vi "DSF.Transceiver.UDP.Tx.vi"(8 "error in (no error)":errorcluster, 9 "Tx":T1, 11 "UDP Transceiver in":refnum<class "DSF.Transceiver.UDP.lvclass">=refnum) -> (0 "error out":errorcluster, 3 "UDP Transceiver out":refnum<class "DSF.Transceiver.UDP.lvclass">)   [LabVIEW 2017, in "DSF.Transceiver.UDP.lvlib" / "DSF.Transceiver.UDP.lvclass"]
uses:
  DSF.Transceiver.UDP.lvclass
  Builds/Current/Data Sharing Framework Core/Data Sharing Framework Core.lvlibp/Engine/Transfer/Transfer.lvclass
  Builds/Current/Data Sharing Framework Core/Data Sharing Framework Core.lvlibp/Engine/Internal/Memory/Memory Buffer/Memory Buffer.lvclass
  Builds/Current/Data Sharing Framework Core/Data Sharing Framework Core.lvlibp/Engine/Internal/Memory/Memory Buffer/Read 1D Array of U8.vi
  DSF.Transceiver.UDP.Parameters.Transfer.Tx.ctl
  DSF.Transceiver.UDP.Parameters.Transfer Group.Tx.ctl
panel:
  in  "Transfers":refnum<class "Transfer.lvclass">[](array[class])
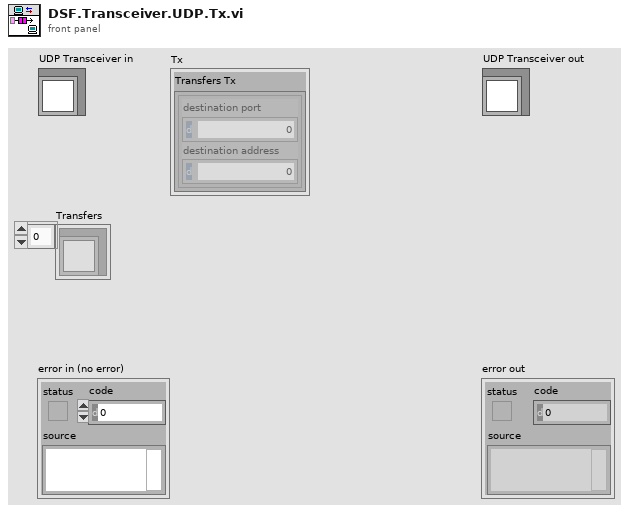
[diagram p1: front panel]
types:
  T1 = typedef "DSF.Transceiver.UDP.lvlib/DSF.Transceiver.UDP.lvclass/DSF.Transceiver.UDP.Parameters.Transfer Group.Tx.ctl" = cluster{"Transfers Tx":T2[]}
  T2 = typedef "DSF.Transceiver.UDP.lvlib/DSF.Transceiver.UDP.lvclass/DSF.Transceiver.UDP.Parameters.Transfer.Tx.ctl" = cluster{"destination port":u16, "destination address":u32}
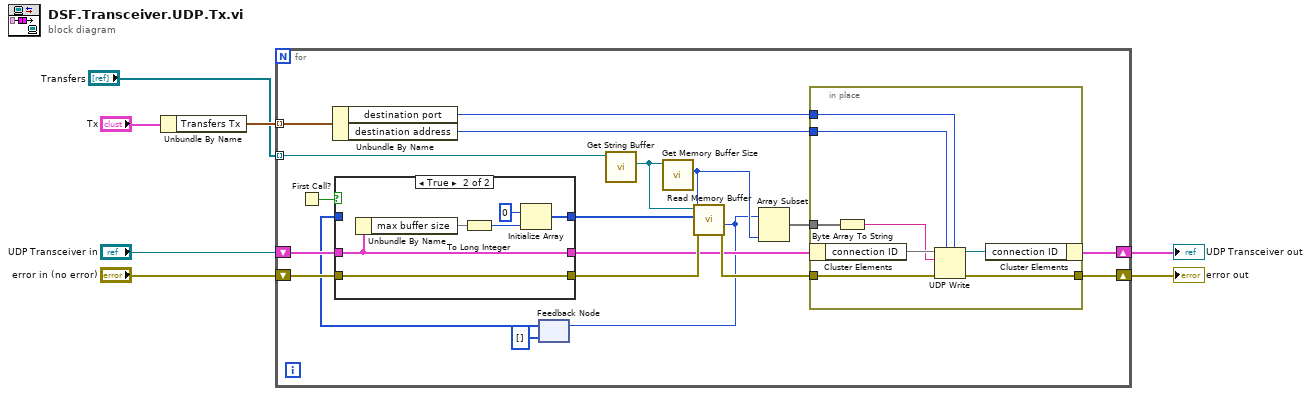
[diagram p0: block diagram]
diagram:
  n1 = Unbundle By Name("Tx") -> ("Transfers Tx"=w2:T2[])
  n2 = for {
    tunnel: "Transfers" -> [w8] mode=indexing
    tunnel: w2 -> [w9] mode=indexing
    shift-right: [w26] -> w7
    shift-left: "error in (no error)" -> [w21]
    shift-right: [w25] -> w6
    shift-left: "UDP Transceiver in" -> [w12]
    n3 = First Call?() -> (First Call?: T/F=w18:bool)
    n4 = Unbundle By Name(w9) -> ("destination port"=w23:u16, "destination address"=w24:u32)
    n5 = feedback #1(u8[] [] ("buffer out")) -> (w11:u8[])
    n6 = case shown="True" w18 {
      tunnel: w12 -> [w28 w34]
      tunnel: w21 -> [w29 w35]
      tunnel: [w29 w35] -> w20
      tunnel: [w28 w34] -> w13
      tunnel: w11 -> [w27 _]
      tunnel: [w27 w31] -> w14
      frame False {
      }
      frame True {
        n7 = Unbundle By Name(w34) -> ("max buffer size"=w33)
        n8 = To Long Integer(number=w33) -> (32bit integer=w30:i32)
        n9 = Initialize Array(u8 0 ("element"), w30) -> (w31:u8[])
      }
    }
    n10 = call "Get String Buffer.vi"("Transfer in"=w8) -> ("Buffer"=w19:refnum<class "Memory Buffer.lvclass">)  [unwired: 9 in, 1 out]
    n11 = call "Get Memory Buffer Size.vi"("Buffer in"=w19) -> ("buffer size"=w17:u64)  [unwired: 9 in, 1 out]
    n12 = call-poly "Read Memory Buffer.vi"("error in (no error)"=w20, "offset (0)"=w17, "buffer in"=w14, "Buffer in"=w19) -> ("error out"=w22:errorcluster, "offset out"=w10:u64)  [unwired: 4 in, 2 out]
    n13 = feedback-in #1(w10) -> ()
    n14 = Array Subset(array=w10, length=w17) -> (w16:void[])  [unwired: 1 in]
    n15 = in-place {
      in-place-border: w22 -> [w43]
      in-place-border: [w40] -> w26
      in-place-border: w24 -> [w39]
      in-place-border: w23 -> [w38]
      in-place-border: w16 -> [w37]
      n16 = in-place-cluster #2(w13) -> ("connection ID"=w42)
      n17 = Byte Array To String(unsigned byte array=w37) -> (string=w36:string)
      n18 = UDP Write(address=w39, port or service name=w38, connection ID=w42, data in=w36, 8:w43) -> (error out=w40:errorcluster, 3:w41:refnum<k16>)  [unwired: 1 in]
      n19 = in-place-cluster #2("connection ID"=w41) -> (w25:cluster{})
    }
  }
  "error out" <- w7
  "UDP Transceiver out" <- w6
